vi "Get_Next_Sub_Collection.vi"(8 "error in (no error)":errorcluster caption="entrée d'erreur (pas d'erreur)", 11 "Firebase AssembledProducts en entrée":refnum<class "Firebase AssembledProducts.lvclass">) -> (0 "error out":errorcluster caption="sortie d'erreur", 3 "Firebase AssembledProducts en sortie":refnum<class "Firebase AssembledProducts.lvclass">)   [LabVIEW 2020, in "Library Instrument & Equipement.lvlib" / "Library FireBase.lvlib" / "Firebase AssembledProducts.lvclass"]
doc: "Return the documents present in the test collection for each DATA read with Get_Data\nPlease initialise the following values\n - Name BDD\n - Document of test sequence\n - API Key\n - Nb To Read"
uses:
  Firebase AssembledProducts.lvclass
  C:/Users/ngarcin/OneDrive - Altyor/Standard TB/Class/Firebase/Source/Firebase Driver/Firebase Driver.lvclass
  Firebase Altyor/Firebase Altyor.lvclass
  Firebase AssembledProducts.lvclass/Firebase AssembledProducts.ctl
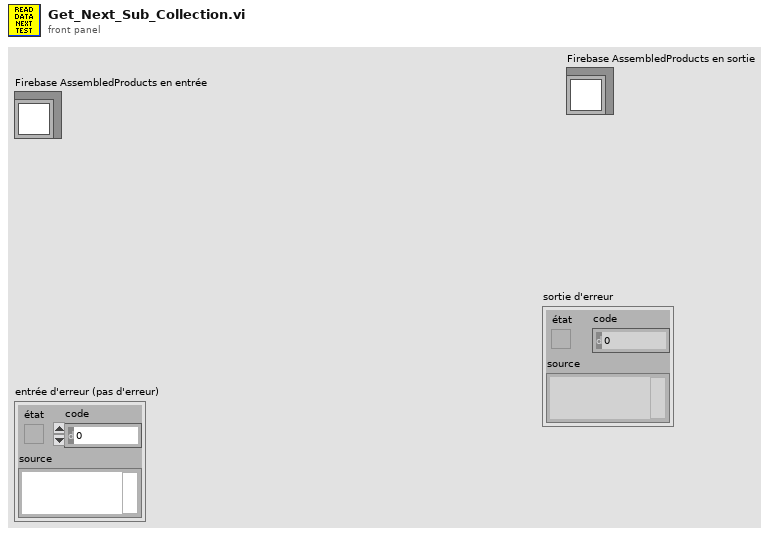
[diagram p1: front panel]
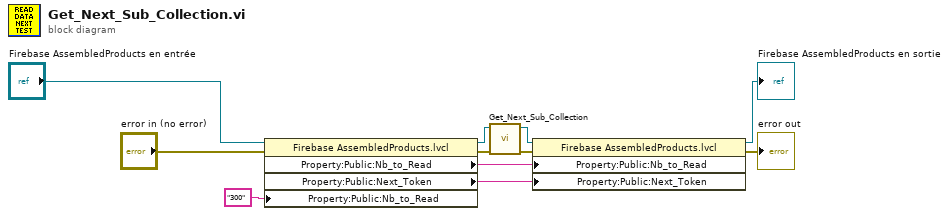
[diagram p0: block diagram]
diagram:
  n1 = property class="Firebase AssembledProducts.lvcl"(reference="Firebase AssembledProducts en entrée", error in="error in (no error)", "Property:Public:Nb_to_Read"="300" ("Nb_to_Read")) -> (reference out=w3:refnum<class "Firebase AssembledProducts.lvclass">, error out=w6:errorcluster, "Property:Public:Nb_to_Read"=w9:string, "Property:Public:Next_Token"=w7:string)
  n2 = call-parent "Get_Next_Sub_Collection.vi"("error in (no error)"=w6, "Firebase Altyor en entrée"=w3) -> ("error out"=w5:errorcluster, "Firebase Altyor en sortie"=w4:refnum<class "Firebase AssembledProducts.lvclass">)  [unwired: 8 in]
  n3 = property class="Firebase AssembledProducts.lvcl"(reference=w4, error in=w5, "Property:Public:Nb_to_Read"=w9, "Property:Public:Next_Token"=w7) -> (reference out=→"Firebase AssembledProducts en sortie":refnum<class "Firebase AssembledProducts.lvclass">, error out=→"error out":errorcluster)
